vi "Write Operator Config.vi"(8 "error in (no error)":errorcluster, 10 "Operator Config":T1, 11 "Operator in":refnum<class "Operator.lvclass">) -> (0 "error out":errorcluster, 3 "Operator out":refnum<class "Operator.lvclass">)   [LabVIEW 2014, in "Operator.lvlib" / "Operator.lvclass"]
uses:
  Operator.lvclass
  Operator Config.ctl
  <vilib>/ActorFramework/Message Enqueuer/Message Enqueuer.lvclass
  Joystick/Joystick Class/Joystick.lvclass
  Operator.lvclass/Operator.ctl
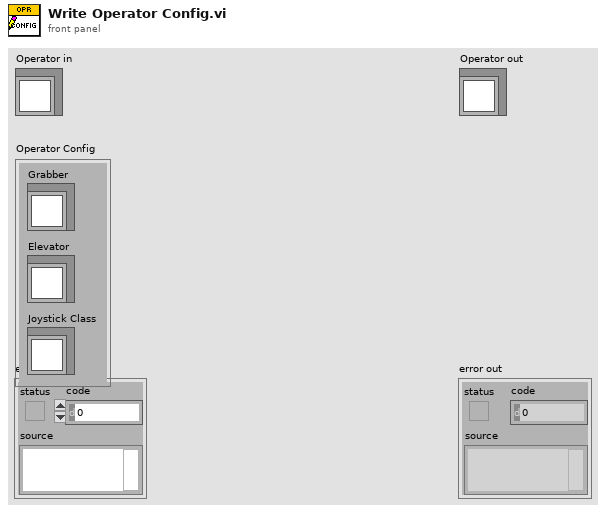
[diagram p1: front panel]
types:
  T1 = typedef "Operator.lvlib/Operator.lvclass/Operator Config.ctl" = cluster{"Grabber":refnum<class "Message Enqueuer.lvclass">, "Joystick Class":refnum<class "Joystick.lvclass">, "Elevator":refnum<class "Message Enqueuer.lvclass">}
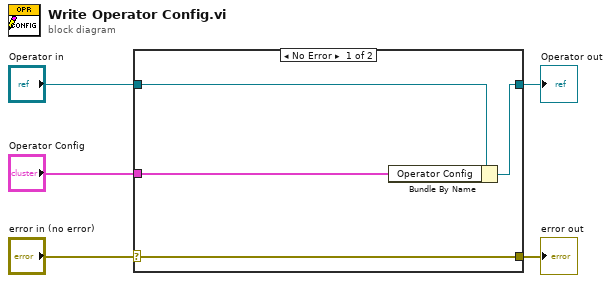
[diagram p0: block diagram]
diagram:
  n1 = case shown="No Error" "error in (no error)" {
    selector: "error in (no error)" -> [w9 w10]
    tunnel: [w9 w10] -> w4
    tunnel: [w7 w11] -> w2
    tunnel: "Operator in" -> [w8 w11]
    tunnel: "Operator Config" -> [w6 _]
    frame No Error {
      n2 = Bundle By Name(cluster=w8, "Operator Config"=w6) -> (w7:refnum<class "Operator.lvclass">)
    }
    frame Error {
    }
  }
  "error out" <- w4
  "Operator out" <- w2
